vi "x502_err_sub.vi"(1 "Error code":i32, 2 "error in (no error)":errorcluster, 3 "Error descr":string) -> (0 "error out":errorcluster)   [LabVIEW 2010]
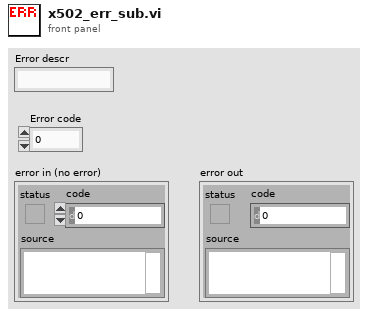
[diagram p1: front panel]
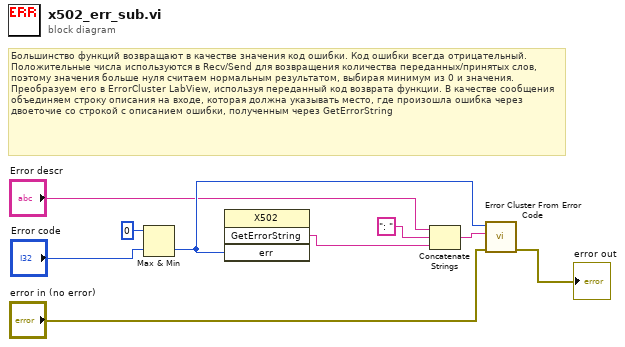
[diagram p0: block diagram]
diagram:
  # "Большинство функций возвращают в качестве значения код ошибки. Код ошибки всегда отрицательный. Положительные числа используются в Recv/Send для возвращения количества переданных/принятых слов, поэтому значения больше нуля считаем нормальным результатом, выбирая минимум из 0 и значения. Преобразуем его в ErrorCluster LabView, используя переданный код возврата функции. В качестве сообщения объединяем строку описания на входе, которая должна указывать место, где произошла ошибка через двоеточие со строкой с описанием ошибки, полученным через GetErrorString"
  n1 = Max & Min(x=0, y="Error code") -> (min(x,y)=w7:i32)  [unwired: 1 out]
  n2 = invoke class="X502" method="GetErrorString"("err"=w7) -> ("GetErrorString"=w1:string)  [unwired: 3 in, 3 out]
  n3 = Concatenate Strings("Error descr", ": ", w1) -> (w9:string)
  n4 = call <vilib>:"Error Cluster From Error Code.vi"("error in (no error)"="error in (no error)", "error message (\"\")"=w9, "error code (0)"=w7) -> ("error out"=→"error out":errorcluster)  [unwired: 6 in]
